vi "Constant Control Panel.vi"(8 "error in (no error)":errorcluster) -> ()   [LabVIEW 2016, in "Constants.lvlib"]
uses:
  Constants.lvlib
  Typedef/Constants.ctl
  <vilib>/Rock Robotics/SystemInterfaces/DIO/FPGA_DIOPWMChannel.ctl
  <vilib>/Rock Robotics/WPI/Joystick/WPI_JoystickDeviceEnum.ctl
  <vilib>/Rock Robotics/SystemInterfaces/DIO/FPGA_DIOChannel.ctl
  <vilib>/Rock Robotics/SystemInterfaces/spilib/spi_bus.ctl
  <vilib>/Rock Robotics/SystemInterfaces/AI/FPGA_AIChannel.ctl
  <vilib>/Rock Robotics/WPI/Solenoid/WPI_SolenoidChannel.ctl
  Private Global.vi
panel:
  out "Written?":bool
  in  "Continuous":bool
  in  "Update Manual":bool
  in  "Constants":T1={"Port Layout"={"RightMotorInverted"=FALSE, "LeftMotorInverted"=TRUE, "Left Motors"=enum."PWM 0", "Right Motors"=enum."PWM 1", "Auton List"=["Alternative 1", "Alternative 2"], "XBOX Port"=enum."USB 0", "Encoder L A"=enum."DIO 3", "Encoder L B"=enum."DIO 4", "Encoder R A"=enum."DIO 5", "Encoder R B"=enum."DIO 6", "L Encoder Inverse"=FALSE, "R Encoder Inverse"=FALSE, "Drive Distance per Count"=0.0, "Gyro Bus"=enum."SPI On-Board, CS2", "Fuel Roller 1"=enum."PWM 0", "Front Roller"=enum."PWM 0", "Gear Flipper"=enum."PWM 0", "Climber 1"=enum."PWM 0", "Fuel Roller Invert"=TRUE, "Front Roller Invert"=TRUE, "Gear Flipper Invert"=TRUE, "Climber Invert"=TRUE, "PCM"=0, "Fuel Roller 2"=enum."PWM 0", "Gear Sensor"=enum."AI 0", "Gear Release Fwd"=enum."Solenoid 0", "Gear Release Rvrs"=enum."Solenoid 0", "Fuel Arm Fwd"=enum."Solenoid 0", "Fuel Arm Rvrs"=enum."Solenoid 0", "Shifter Fwrd"=enum."Solenoid 0", "Shifter Rvrs"=enum."Solenoid 0", "Climber 2"=enum."PWM 0", "PDP"=60, "Shooter Front Channel"=0, "Shooter Rear Channel"=0, "Shooter Feed Channel"=0, "Camera Servo"=enum."PWM 0", "Gear Servo"=enum."PWM 0", "Gear Puncher Fwrd"=enum."Solenoid 0", "Gear Puncher Rvrs"=enum."Solenoid 0", "Shooter Inverse"=TRUE, "Ring Light Switch"=enum."DIO 4"}, "Drive Constants"={"Wheelbase In."=1.0, "Max Velocity (In/sec)"=78.0, "Max Accel (In/sec^2)"=78.0, "Max Jerk (In/sec^3)"=0.0, "Path dt"=0.0, "Path Sample Count"=0, "Deadband"=0.35}, "Arm System"={"Front Roller Gear Speed"=0.8, "Front Roller Fuel Speed"=0.8, "Gear Flipper Speed"=0.8, "Fuel Roller Speed"=0.8, "Gear Release Wait (ms)"=1000, "Gear Sensor Threshold"=0.3, "Flappy Open Angle"=0, "Flappy Close Angle"=0, "Ramp Rate (EGU/min)"=200.0}, "Shooter"={"Shooter Wheels"={"P"=0.0, "I"=0.0, "D"=0.0, "F"=0.0, "IZone"=0.0}, "Feeder"={"P"=0.0, "I"=0.0, "D"=0.0, "F"=0.0, "IZone"=0.0}, "Front Shooter RPM"=0.0, "Rear Shooter RPM"=0.0, "Agitator Speed"=0.0, "Feeder Speed"=0.0, "Shooter CPR"=0, "Feeder CPR"=0}, "Vision"={"High Goal Height (in.)"=0.0, "Low Goal Height (in.)"=0.0, "Camera Height High (in.)"=0.0, "Camera Height Low (in.)"=0.0, "Servo Pitch Gear (deg)"=0.0, "Camera Yaw (deg)"=0.0, "Servo Gear"=0, "Servo Boiler"=0, "Servo Pitch Boiler (deg)"=0.0}}
  in  "file":path=path "/home/lvuser/constants.xml"
  in  "Write File":bool
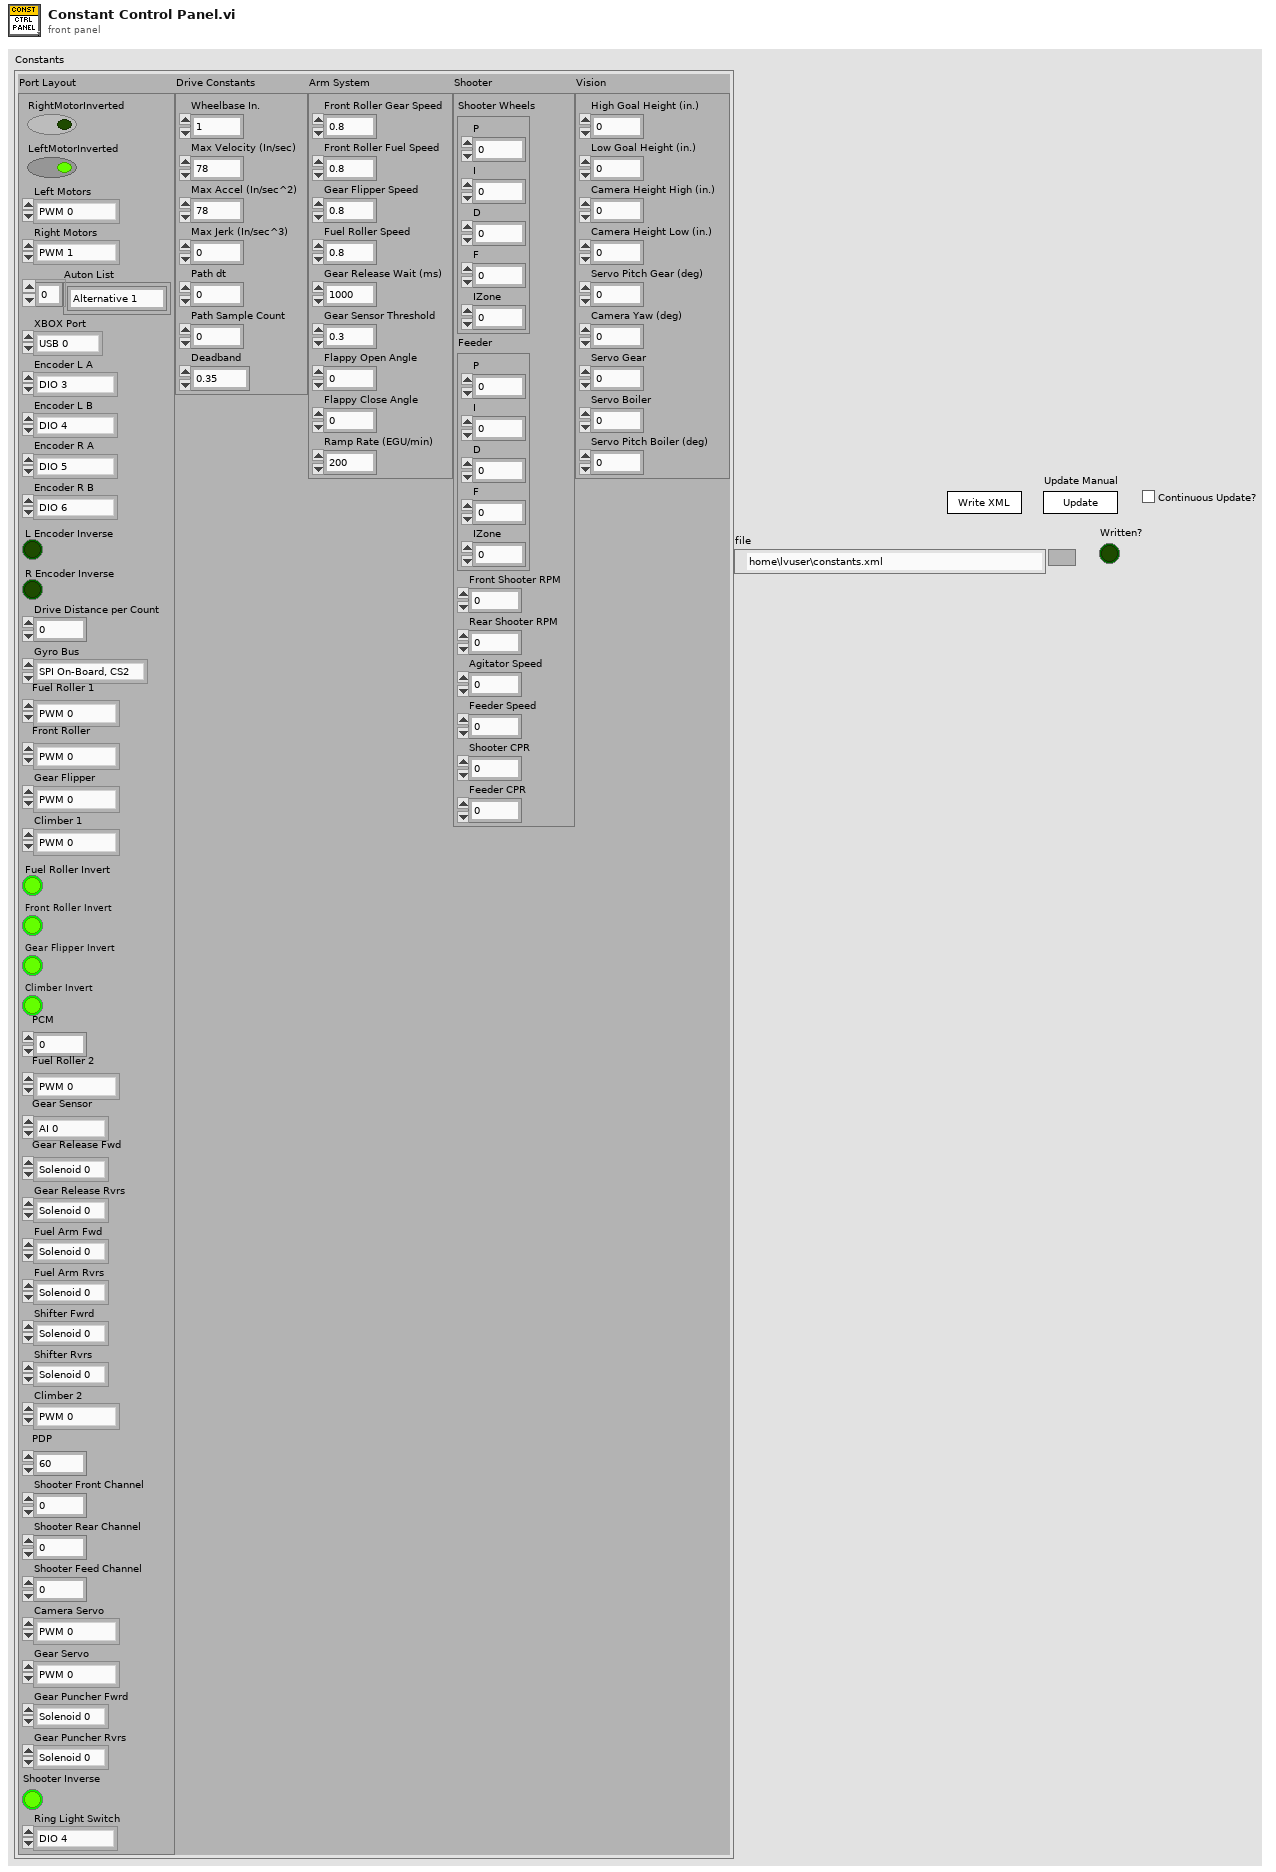
[diagram p1: front panel]
types:
  T1 = typedef "Constants.lvlib/Constants.ctl" = cluster{"Port Layout":cluster{"RightMotorInverted":bool, "LeftMotorInverted":bool, "Left Motors":T2, "Right Motors":T2, "Auton List":string[], "XBOX Port":T3, "Encoder L A":T4, "Encoder L B":T4, "Encoder R A":T4, "Encoder R B":T4, "L Encoder Inverse":bool, "R Encoder Inverse":bool, "Drive Distance per Count":dbl, "Gyro Bus":T5, "Fuel Roller 1":T2, "Front Roller":T2, "Gear Flipper":T2, "Climber 1":T2, "Fuel Roller Invert":bool, "Front Roller Invert":bool, "Gear Flipper Invert":bool, "Climber Invert":bool, "PCM":u8, "Fuel Roller 2":T2, "Gear Sensor":T6, "Gear Release Fwd":T7, "Gear Release Rvrs":T7, "Fuel Arm Fwd":T7, "Fuel Arm Rvrs":T7, "Shifter Fwrd":T7, "Shifter Rvrs":T7, "Climber 2":T2, "PDP":u8, "Shooter Front Channel":u8, "Shooter Rear Channel":u8, "Shooter Feed Channel":u8, "Camera Servo":T2, "Gear Servo":T2, "Gear Puncher Fwrd":T7, "Gear Puncher Rvrs":T7, "Shooter Inverse":bool, "Ring Light Switch":T4}, "Drive Constants":cluster{"Wheelbase In.":dbl, "Max Velocity (In/sec)":dbl, "Max Accel (In/sec^2)":dbl, "Max Jerk (In/sec^3)":dbl, "Path dt":dbl, "Path Sample Count":i32, "Deadband":dbl}, "Arm System":cluster{"Front Roller Gear Speed":dbl, "Front Roller Fuel Speed":dbl, "Gear Flipper Speed":dbl, "Fuel Roller Speed":dbl, "Gear Release Wait (ms)":i32, "Gear Sensor Threshold":dbl, "Flappy Open Angle":i32, "Flappy Close Angle":i32, "Ramp Rate (EGU/min)":dbl}, "Shooter":cluster{"Shooter Wheels":cluster{"P":dbl, "I":dbl, "D":dbl, "F":dbl, "IZone":dbl}, "Feeder":cluster{"P":dbl, "I":dbl, "D":dbl, "F":dbl, "IZone":dbl}, "Front Shooter RPM":dbl, "Rear Shooter RPM":dbl, "Agitator Speed":dbl, "Feeder Speed":dbl, "Shooter CPR":u32, "Feeder CPR":u32}, "Vision":cluster{"High Goal Height (in.)":dbl, "Low Goal Height (in.)":dbl, "Camera Height High (in.)":dbl, "Camera Height Low (in.)":dbl, "Servo Pitch Gear (deg)":dbl, "Camera Yaw (deg)":dbl, "Servo Gear":i32, "Servo Boiler":i32, "Servo Pitch Boiler (deg)":dbl}}
  T2 = typedef "FPGA_DIOPWMChannel.ctl" = enum8{"PWM 0", "PWM 1", "PWM 2", "PWM 3", "PWM 4", "PWM 5", "PWM 6", "PWM 7", "PWM 8", "PWM 9", "PWM MXP 0", "PWM MXP 1", "PWM MXP 2", "PWM MXP 3", "PWM MXP 4", "PWM MXP 5", "PWM MXP 6", "PWM MXP 7", "PWM MXP 8", "PWM MXP 9", "Invalid"}
  T3 = typedef "WPI_JoystickDeviceEnum.ctl" = enum16{"USB 0", "USB 1", "USB 2", "USB 3", "USB 4", "USB 5"}
  T4 = typedef "FPGA_DIOChannel.ctl" = enum8{"DIO 0", "DIO 1", "DIO 2", "DIO 3", "DIO 4", "DIO 5", "DIO 6", "DIO 7", "DIO 8", "DIO 9", "DIO MXP 0", "DIO MXP 1", "DIO MXP 2", "DIO MXP 3", "DIO MXP 4", "DIO MXP 5", "DIO MXP 6", "DIO MXP 7", "DIO MXP 8", "DIO MXP 9", "DIO MXP 10", "DIO MXP 11", "DIO MXP 12", "DIO MXP 13", "DIO MXP 14", "DIO MXP 15", "SPI Port CS1", "SPI Port CS2", "SPI Port CS3", "SPI Port MISO", "SPI Port MOSI", "Invalid"}
  T5 = typedef "spi_bus.ctl" = enum16{"SPI On-Board, CS0", "SPI On-Board, CS1", "SPI On-Board, CS2", "SPI On-Board, CS3", "SPI MXP", "Invalid"}
  T6 = typedef "FPGA_AIChannel.ctl" = enum8{"AI 0", "AI 1", "AI 2", "AI 3", "AI MXP 0", "AI MXP 1", "AI MXP 2", "AI MXP 3", "Invalid"}
  T7 = typedef "WPI_SolenoidChannel.ctl" = enum8{"Solenoid 0", "Solenoid 1", "Solenoid 2", "Solenoid 3", "Solenoid 4", "Solenoid 5", "Solenoid 6", "Solenoid 7", "Invalid"}
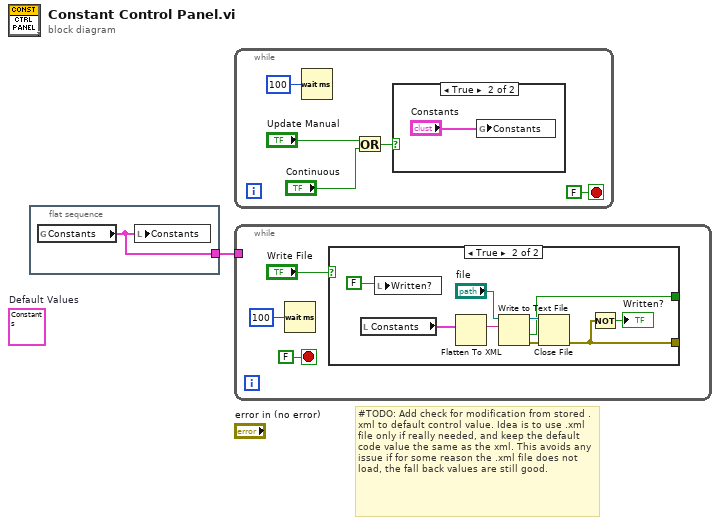
[diagram p0: block diagram]
diagram:
  (unwired) T1 {"Port Layout"={"RightMotorInverted"=FALSE, "LeftMotorInverted"=TRUE, "Left Motors"=enum."PWM 0", "Right Motors"=enum."PWM 1", "Auton List"=["Alternative 1", "Alternative 2"], "XBOX Port"=enum."USB 0", "Encoder L A"=enum."DIO 3", "Encoder L B"=enum."DIO 4", "Encoder R A"=enum."DIO 5", "Encoder R B"=enum."DIO 6", "L Encoder Inverse"=FALSE, "R Encoder Inverse"=FALSE, "Drive Distance per Count"=0.0, "Gyro Bus"=enum."SPI On-Board, CS2", "Fuel Roller 1"=enum."PWM 0", "Front Roller"=enum."PWM 0", "Gear Flipper"=enum."PWM 0", "Climber 1"=enum."PWM 0", "Fuel Roller Invert"=TRUE, "Front Roller Invert"=TRUE, "Gear Flipper Invert"=TRUE, "Climber Invert"=TRUE, "PCM"=0, "Fuel Roller 2"=enum."PWM 0", "Gear Sensor"=enum."AI 0", "Gear Release Fwd"=enum."Solenoid 0", "Gear Release Rvrs"=enum."Solenoid 0", "Fuel Arm Fwd"=enum."Solenoid 0", "Fuel Arm Rvrs"=enum."Solenoid 0", "Shifter Fwrd"=enum."Solenoid 0", "Shifter Rvrs"=enum."Solenoid 0", "Climber 2"=enum."PWM 0", "PDP"=60, "Shooter Front Channel"=0, "Shooter Rear Channel"=0, "Shooter Feed Channel"=0, "Camera Servo"=enum."PWM 0", "Gear Servo"=enum."PWM 0", "Gear Puncher Fwrd"=enum."Solenoid 0", "Gear Puncher Rvrs"=enum."Solenoid 0", "Shooter Inverse"=TRUE, "Ring Light Switch"=enum."DIO 4"}, "Drive Constants"={"Wheelbase In."=1.0, "Max Velocity (In/sec)"=78.0, "Max Accel (In/sec^2)"=78.0, "Max Jerk (In/sec^3)"=0.0, "Path dt"=0.0, "Path Sample Count"=0, "Deadband"=0.35}, "Arm System"={"Front Roller Gear Speed"=0.8, "Front Roller Fuel Speed"=0.8, "Gear Flipper Speed"=0.8, "Fuel Roller Speed"=0.8, "Gear Release Wait (ms)"=1000, "Gear Sensor Threshold"=0.3, "Flappy Open Angle"=0, "Flappy Close Angle"=0, "Ramp Rate (EGU/min)"=200.0}, "Shooter"={"Shooter Wheels"={"P"=0.0, "I"=0.0, "D"=0.0, "F"=0.0, "IZone"=0.0}, "Feeder"={"P"=0.0, "I"=0.0, "D"=0.0, "F"=0.0, "IZone"=0.0}, "Front Shooter RPM"=0.0, "Rear Shooter RPM"=0.0, "Agitator Speed"=0.0, "Feeder Speed"=0.0, "Shooter CPR"=0, "Feeder CPR"=0}, "Vision"={"High Goal Height (in.)"=0.0, "Low Goal Height (in.)"=0.0, "Camera Height High (in.)"=0.0, "Camera Height Low (in.)"=0.0, "Servo Pitch Gear (deg)"=0.0, "Camera Yaw (deg)"=0.0, "Servo Gear"=0, "Servo Boiler"=0, "Servo Pitch Boiler (deg)"=0.0}}  # Default Values
  # "#TODO: Add check for modification from stored .xml to default control value. Idea is to use .xml file only if really needed, and keep the default code value the same as the xml. This avoids any issue if for some reason the .xml file does not load, the fall back values are still good."
  n1 = flat-sequence {
    tunnel: [w2] -> w1
    frame #0 {
      n2 = global read "Private Global.vi" "Constants"() -> (w2:T1)
      n3 = local write "Constants"(w2) -> ()
    }
  }
  n4 = while {
    stop <- FALSE stop-if-true
    n5 = Wait (ms)(milliseconds to wait=u32 100) -> ()  [unwired: 1 out]
    n6 = Or(x="Update Manual", y="Continuous") -> (x .or. y?=w4:bool)
    n7 = case shown="True" w4 {
      frame False {
      }
      frame True {
        n8 = global write "Private Global.vi" "Constants"("Constants") -> ()
      }
    }
  }
  n9 = while {
    tunnel: w1 -> [_]
    stop <- FALSE stop-if-true
    n10 = Wait (ms)(milliseconds to wait=u32 100) -> ()  [unwired: 1 out]
    n11 = case shown="True" "Write File" {
      tunnel: [_ w13] -> _
      tunnel: [_ w16] -> _
      frame False {
      }
      frame True {
        n12 = local read "Constants"() -> (w15:T1)
        n13 = local write "Written?"(FALSE) -> ()
        n14 = Flatten To XML(anything=w15) -> (xml string=w19:string)
        n15 = Write to Text File(file (use dialog)="file", text=w19) -> (refnum out=w17:refnum<file>, cancelled=w16:bool, error out=w18:errorcluster)  [unwired: 2 in]
        n16 = Close File(refnum=w17, error in=w18) -> (error out=w13:errorcluster)  [unwired: 1 out]
        n17 = Not(x=w13) -> (.not. x?=→"Written?":bool)
      }
    }
  }
